vi "tap_with_light_pulse.vi"() -> ()   [LabVIEW 2019]
panel:
  in  "Hold light before tap (frames)":dbl
  in  "Stimuli duration (frames)":dbl
  in  "Period (blank+sti)(frames)":dbl
  in  "Light power (uW/mm^2)":i32
  in  "Taps per stimulus (count)":i32
  in  "Total duration (frames)":dbl
  out "Frames":i32
  in  "Transfer and Run Date Folder After Experiment":bool
  in  "SSH user name":string
  in  "SSH password":string
  in  "Wait before recording (s)":dbl
  in  "Tags":string
  in  "Start Recording":bool
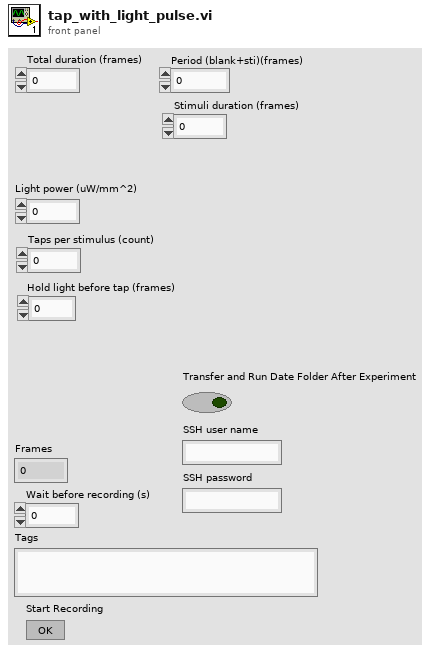
[diagram p1: front panel]
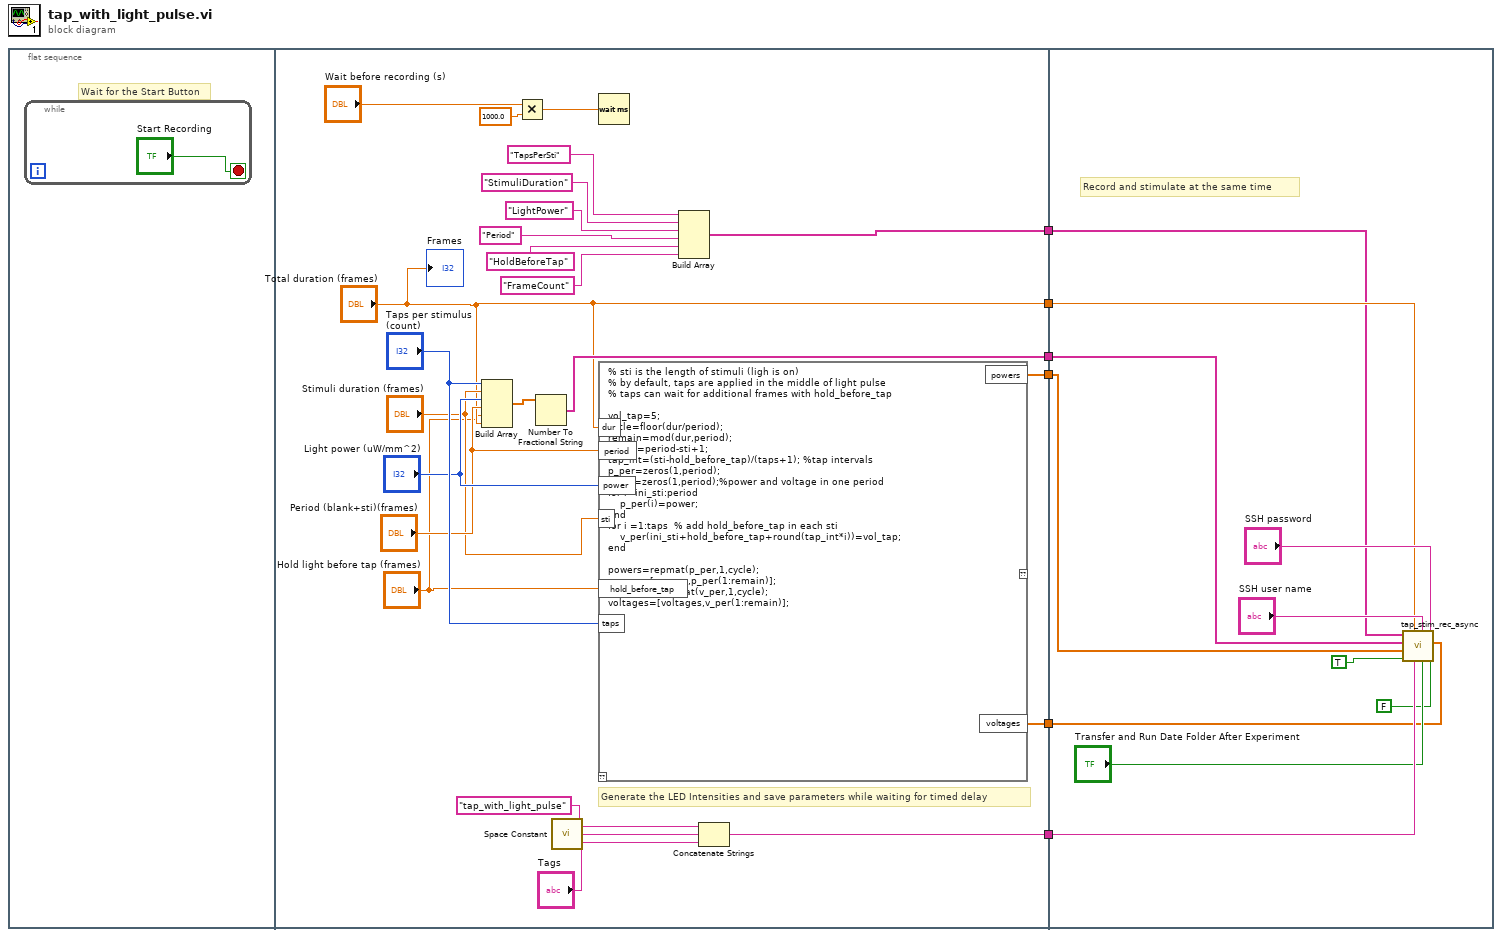
[diagram p0: block diagram]
diagram:
  n1 = flat-sequence {
    tunnel: [w28] -> w6
    tunnel: [w19] -> w5
    tunnel: ["Total duration (frames)"] -> w4
    tunnel: [w17] -> w3
    tunnel: [w13] -> w2
    tunnel: [w12] -> w1
    tunnel: w6 -> [w42]
    tunnel: w5 -> [w34]
    tunnel: w4 -> [w38]
    tunnel: w3 -> [w37]
    tunnel: w2 -> [w33]
    tunnel: w1 -> [w32]
    frame #0 {
      # "Wait for the Start Button"
      n2 = while {
        stop <- "Start Recording" stop-if-true
      }
    }
    frame #1 {
      # "Generate the LED Intensities and save parameters while waiting for timed delay"
      n3 = Build Array("Taps per stimulus (count)", "Stimuli duration (frames)", "Light power (uW/mm^2)", "Period (blank+sti)(frames)", "Hold light before tap (frames)", "Total duration (frames)") -> (w18:dbl[])
      n4 = Multiply(x="Wait before recording (s)", y=1000.0) -> (x*y=w26:dbl)
      n5 = Number To Fractional String(number=w18) -> (F-format string=w12:string[])  [unwired: 3 in]
      n6 = call <vilib>:"Space Constant.vi"() -> ("String"=w30:string)
      n7 = Wait (ms)(milliseconds to wait=w26) -> ()  [unwired: 1 out]
      n8 = script code="% sti is the length of stimuli (ligh is on)\n% by default, taps are applied in the middle of light pulse\n% taps can wait for additional frames with hold_before_tap\n\nvol_tap=5;\ncycle=floor(dur/period);\nremain=mod(dur,period);\nini_sti=period-sti+1;\ntap_int=(sti-hold_before_tap)/(taps+1); %tap intervals\np_per=zeros(1,period);\nv_per=zeros(1,period);%power and voltage in one period\nfor i=ini_sti:period  \n    p_per(i)=power;\nend\nfor i =1:taps  % add hold_before_tap in each sti\n    v_per(ini_sti+hold_before_tap+round(tap_int*i))=vol_tap; \nend\n\npowers=repmat(p_per,1,cycle);\npowers=[powers,p_per(1:remain)];\nvoltages =repmat(v_per,1,cycle);\nvoltages=[voltages,v_per(1:remain)];"("power"="Light power (uW/mm^2)", "taps"="Taps per stimulus (count)", "sti"="Stimuli duration (frames)", "period"="Period (blank+sti)(frames)", "dur"="Total duration (frames)", "hold_before_tap"="Hold light before tap (frames)") -> ("powers"=w17:dbl[], "voltages"=w13:dbl[])  [unwired: 1 in, 1 out]
      n9 = Build Array("TapsPerSti", "StimuliDuration", "LightPower", "Period", "HoldBeforeTap", "FrameCount") -> (w19:string[])
      n10 = Concatenate Strings("tap_with_light_pulse", w30, "Tags") -> (w28:string)
      "Frames" <- "Total duration (frames)"
    }
    frame #2 {
      # "Record and stimulate at the same time"
      n11 = call "tap_stim_rec_async.vi"("Convert Power to Voltage B"=FALSE, "voltages/power B"=w33, "SSH password"="SSH password", "Transfer and Run Date Folder After Experiment"="Transfer and Run Date Folder After Experiment", "SSH user name"="SSH user name", "Tags"=w42, "Frames"=w38, "Convert Power to Voltage A"=TRUE, "voltages/power A"=w37, "parameters"=w32, "parameters headers"=w34) -> ()  [unwired: 1 in]
    }
  }
